vi "write8.vi"(8 "error out":errorcluster caption="error in", 9 "起始地址":u32, 10 "数组":u8[](array[numeric]), 11 "VISA资源名称输入":refnum<visa-resource-name>) -> (0 "error out 2":errorcluster caption="error out", 3 "VISA资源名称 输出":refnum<visa-resource-name>)   [LabVIEW 2012]
uses:
  <vilib>/Instr/_visa.llb/VISA Register Access Address Space.ctl
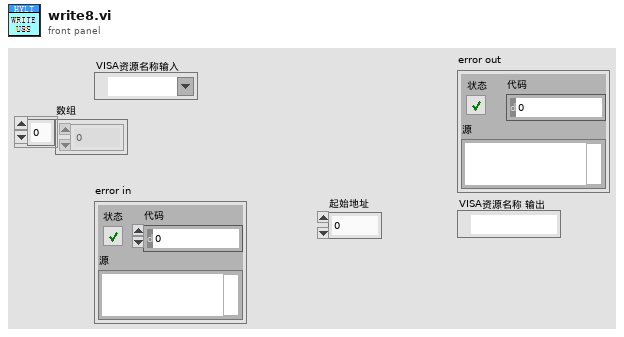
[diagram p1: front panel]
types:
  T1 = typedef "VISA Register Access Address Space.ctl" = u16
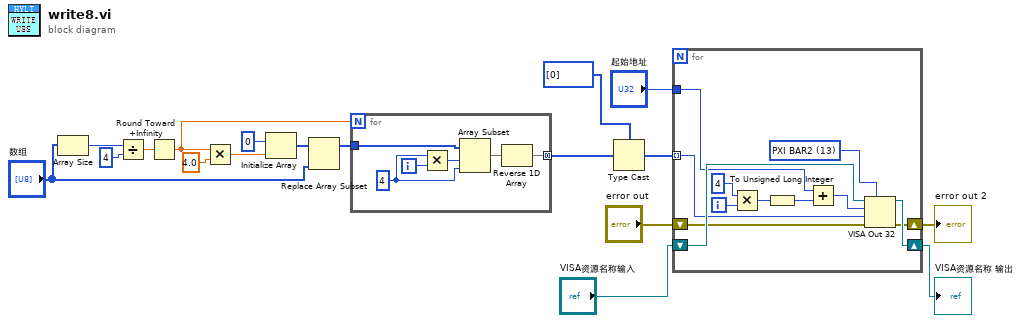
[diagram p0: block diagram]
diagram:
  n1 = Array Size(array="数组") -> (size(s)=w10:i32)
  n2 = Divide(x=w10, y=4) -> (x/y=w12:dbl)
  n3 = Round Toward +Infinity(x=w12) -> (ceil(x): smallest int >= x=w8:dbl)
  n4 = Multiply(x=w8, y=4.0) -> (x*y=w6:dbl)
  n5 = Initialize Array(u8 0 ("元素"), w6) -> (w4:u8[])
  n6 = Replace Array Subset(array=w4, new element="数组") -> (w3:u8[])  [unwired: 1 in]
  n7 = for {
    N: w8 -> [_]
    tunnel: w3 -> [w24]
    tunnel: [w19] -> w9 mode=concatenating
    i -> [w23]
    w21 = 4 ("x")
    n8 = Multiply(x=w21, y=w23) -> (x*y=w22:i32)
    n9 = Array Subset(array=w24, index=w22, length=w21) -> (w20:u8[])
    n10 = Reverse 1D Array(array=w20) -> (reversed array=w19:u8[])
  }
  n11 = Type Cast(type=u32[] [0], x=w9) -> (*(type *) &x=w1:u32[])
  n12 = for {
    tunnel: w1 -> [w26] mode=indexing
    tunnel: "起始地址" -> [w35]
    shift-right: [w32] -> w15
    shift-left: "VISA资源名称输入" -> [w36]
    shift-right: [w31] -> w16
    shift-left: "error out" -> [w30]
    i -> [w34]
    w27 = T1 13 items=["VXI/VME A16"=1, "VXI/VME A24"=2, "VXI/VME A32"=3, "VXI/VME A64"=4, "PXI内存分配"=9, "PXI配置"=10, "PXI BAR0"=11, "PXI BAR1"=12, "PXI BAR2"=13, "PXI BAR3"=14, "PXI BAR4"=15, "PXI BAR5"=16] ("Address Space")
    n13 = Multiply(x=4, y=w34) -> (x*y=w29:i32)
    n14 = To Unsigned Long Integer(number=w29) -> (unsigned 32bit integer=w25:u32)
    n15 = Add(x=w35, y=w25) -> (x+y=w28:u32)
    n16 = VISA Out 32(7:w27, 8:w30, 9:w26, 10:w28, 11:w36) -> (0:w31:errorcluster, 3:w32:refnum<visa-resource-name>)
  }
  "error out 2" <- w16
  "VISA资源名称 输出" <- w15
